vi "ZK仪器状态.vi"(8 "error in (no error)":errorcluster, 11 "Slave ID":T3) -> (0 "error out":errorcluster, 2 "质控仪器状态显示":T1, 3 "质控仪器状态":T2 {"当前步骤数" format="0x%04xH"})   [LabVIEW 2016, in "质控单元V4.lvlib"]
uses:
  <vilib>/Plasmionique/MB Master/MB_Master/MB_Master.lvclass
  <vilib>/Plasmionique/MB Master/MB Master.lvlib
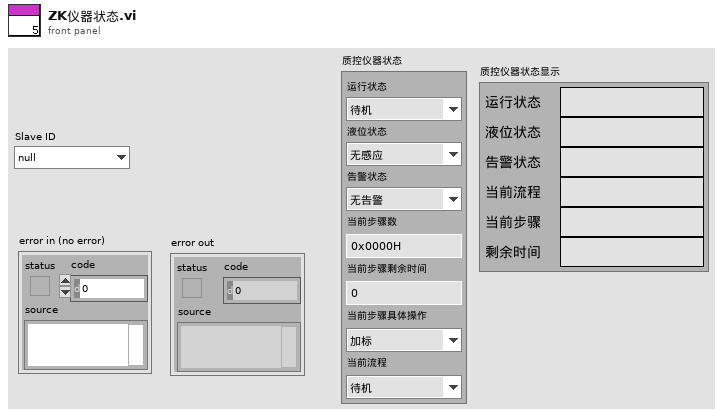
[diagram p1: front panel]
types:
  T1 = typedef "质控单元V4.lvlib/质控仪器状态显示.ctl" = cluster{"运行状态":string, "液位状态":string, "告警状态":string, "当前流程":string, "当前步骤":string, "剩余时间":string}
  T2 = typedef "质控单元V4.lvlib/质控仪器状态.ctl" = cluster{"运行状态":enum16{"待机", "润洗", "进样", "定量", "加标", "等待取样", "排液", "异常停机"}, "液位状态":enum16{"无感应", "有感应"}, "告警状态":enum16{"无告警", "液位故障告警", "注射泵异常"}, "当前步骤数":u16, "当前步骤剩余时间":u16, "当前步骤具体操作":enum16{"加标", "进样", "排液", "搅拌", "定量"}, "当前流程":enum16{"待机", "进样流程", "加标流程", "排液流程", "润洗流程"}}
  T3 = typedef "质控单元V4.lvlib/质控slave id.ctl" = enum16{"null", "氨氮", "总磷", "总氮", "CODMn", "CODCr", "氨氮总磷", "总磷总氮"}
  T4 = cluster{"[0]":u16, "[1]":u16, "[2]":u16, "[3]":u16, "[4]":u16, "[5]":u16, "[6]":u16}
  T5 = cluster{"RingText.Text":string, "RingText.Text":string, "RingText.Text":string, string, "RingText.Text":string, string}
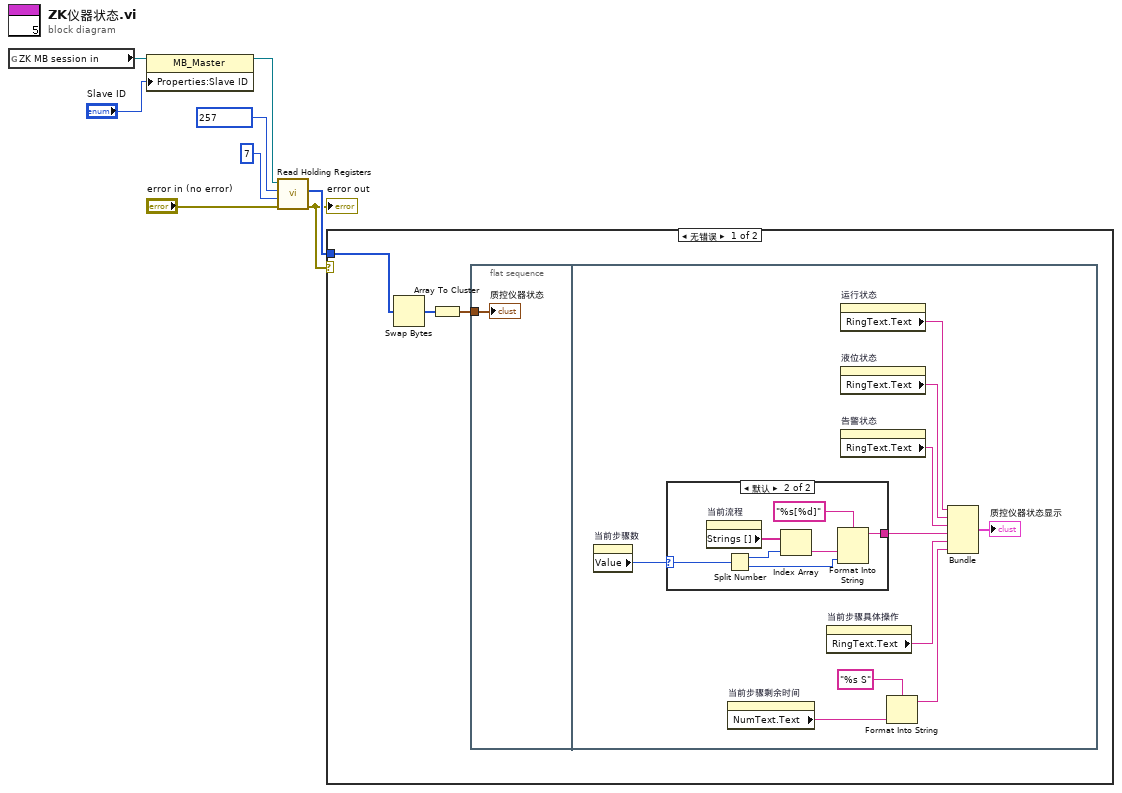
[diagram p0: block diagram]
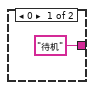
[diagram p2: hidden frame]
diagram:
  n1 = global read "ZK非断电保存全局变量.vi" "ZK MB session in"() -> (w7:refnum<class "MB_Master.lvclass">)
  n2 = property class="MB_Master"(reference=w7, "Properties:Slave ID"="Slave ID") -> (reference out=w5:refnum<class "MB_Master.lvclass">)  [unwired: 1 in, 1 out]
  n3 = call <vilib>:"Read Holding Registers.vi"("error in (no error)"="error in (no error)", "quantity"=u16 7, "starting address"=u16 257, "MB session in"=w5) -> ("error out"=w1:errorcluster, "Registers"=w2:u16[])  [unwired: 5 in, 1 out]
  "error out" <- w1
  n4 = case shown="无错误" w1 {
    tunnel: w2 -> [w11 _]
    frame No Error {
      n5 = Swap Bytes(anything=w11) -> (byte swapped=w10:u16[])
      n6 = Array To Cluster(array=w10) -> (cluster=w9:T4)
      n7 = flat-sequence {
        tunnel: w9 -> [w12]
        frame #0 {
          "质控仪器状态" <- w12
        }
        frame #1 {
          n8 = property on="当前步骤数" class="DigNum (严格)"() -> ("Value"=w14:u16)  [unwired: 2 in, 2 out]
          n9 = case shown="默认" w14 {
            selector: w14 -> [_ w24]
            tunnel: ["待机" w25] -> w19
            frame 0 {
            }
            frame Default {
              n10 = property on="当前流程" class="Enum (严格)"() -> ("Strings []"=w28:string[])  [unwired: 2 in, 2 out]
              n11 = Split Number(x=w24) -> (hi(x)=w29:u8, lo(x)=w27:u8)
              n12 = Index Array(array=w28, index=w29) -> (element=w30:string)
              n13 = Format Into String(format string="%s[%d]" ("格式字符串"), w30, w27) -> (resulting string=w25:string)  [unwired: 2 in, 1 out]
            }
          }
          n14 = property on="当前步骤剩余时间" class="DigNum (严格)"() -> ("NumText.Text"=w16:string)  [unwired: 2 in, 2 out]
          n15 = property on="当前步骤具体操作" class="Enum (严格)"() -> ("RingText.Text"=w18:string)  [unwired: 2 in, 2 out]
          n16 = property on="运行状态" class="Enum (严格)"() -> ("RingText.Text"=w22:string)  [unwired: 2 in, 2 out]
          n17 = property on="液位状态" class="Enum (严格)"() -> ("RingText.Text"=w21:string)  [unwired: 2 in, 2 out]
          n18 = property on="告警状态" class="Enum (严格)"() -> ("RingText.Text"=w20:string)  [unwired: 2 in, 2 out]
          n19 = Format Into String(format string="%s S" ("格式字符串"), w16) -> (resulting string=w15:string)  [unwired: 2 in, 1 out]
          n20 = Bundle("RingText.Text"=w22, "RingText.Text"=w21, "RingText.Text"=w20, w19, "RingText.Text"=w18, w15) -> (→"质控仪器状态显示":T5)  [unwired: 1 in]
        }
      }
    }
    frame Error {
    }
  }
